vi "CRYResult save as text.vi"(4 "File exists & overwrite (F)":bool, 5 "Excel path":path, 6 "Comment":string, 7 "New/Append":string, 8 "File format":u32, 9 "Format info":T1, 10 "Path":path, 11 "Results stack, flat":string[](array[string])) -> ()   [LabVIEW 2013]
uses:
  Data/CRYData & result stacks global.vi
panel:
  out "error out":errorcluster
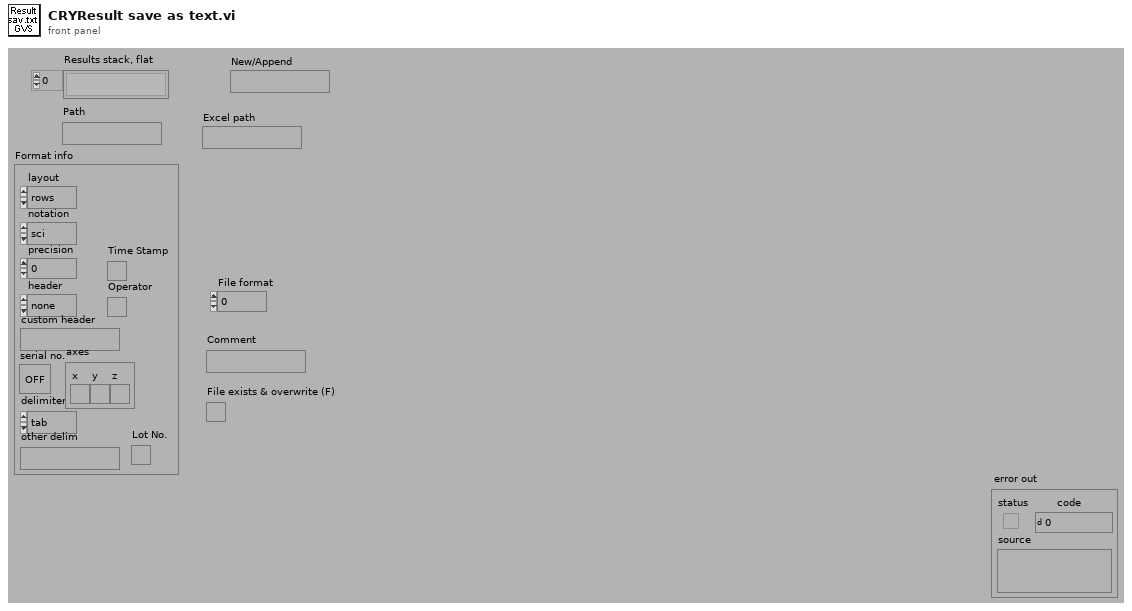
[diagram p1: front panel]
types:
  T1 = cluster{"layout":enum16{"rows", "columns"}, "notation":enum16{"sci", "float"}, "precision":i32, "header":enum16{"none", "standard", "custom"}, "custom header":string, "serial no.":bool, "delimiter":enum16{"tab", "comma", "space", "other"}, "other delim":string, "axes":cluster{"x":bool, "y":bool, "z":bool}, "Lot No.":bool, "Operator":bool, "Time Stamp":bool}
  T2 = typedef "CRYResult Cluster.ctl" = cluster{"Name":string, "Margin":dbl, "unit":string, "Verdict":bool, "Limit":string, "Max/Min":string, "protected":bool, "Step No.":i32, "Test Info":string, "AutoProtect":bool}
  T3 = enum16{"open", "open or create", "create or replace", "create"}
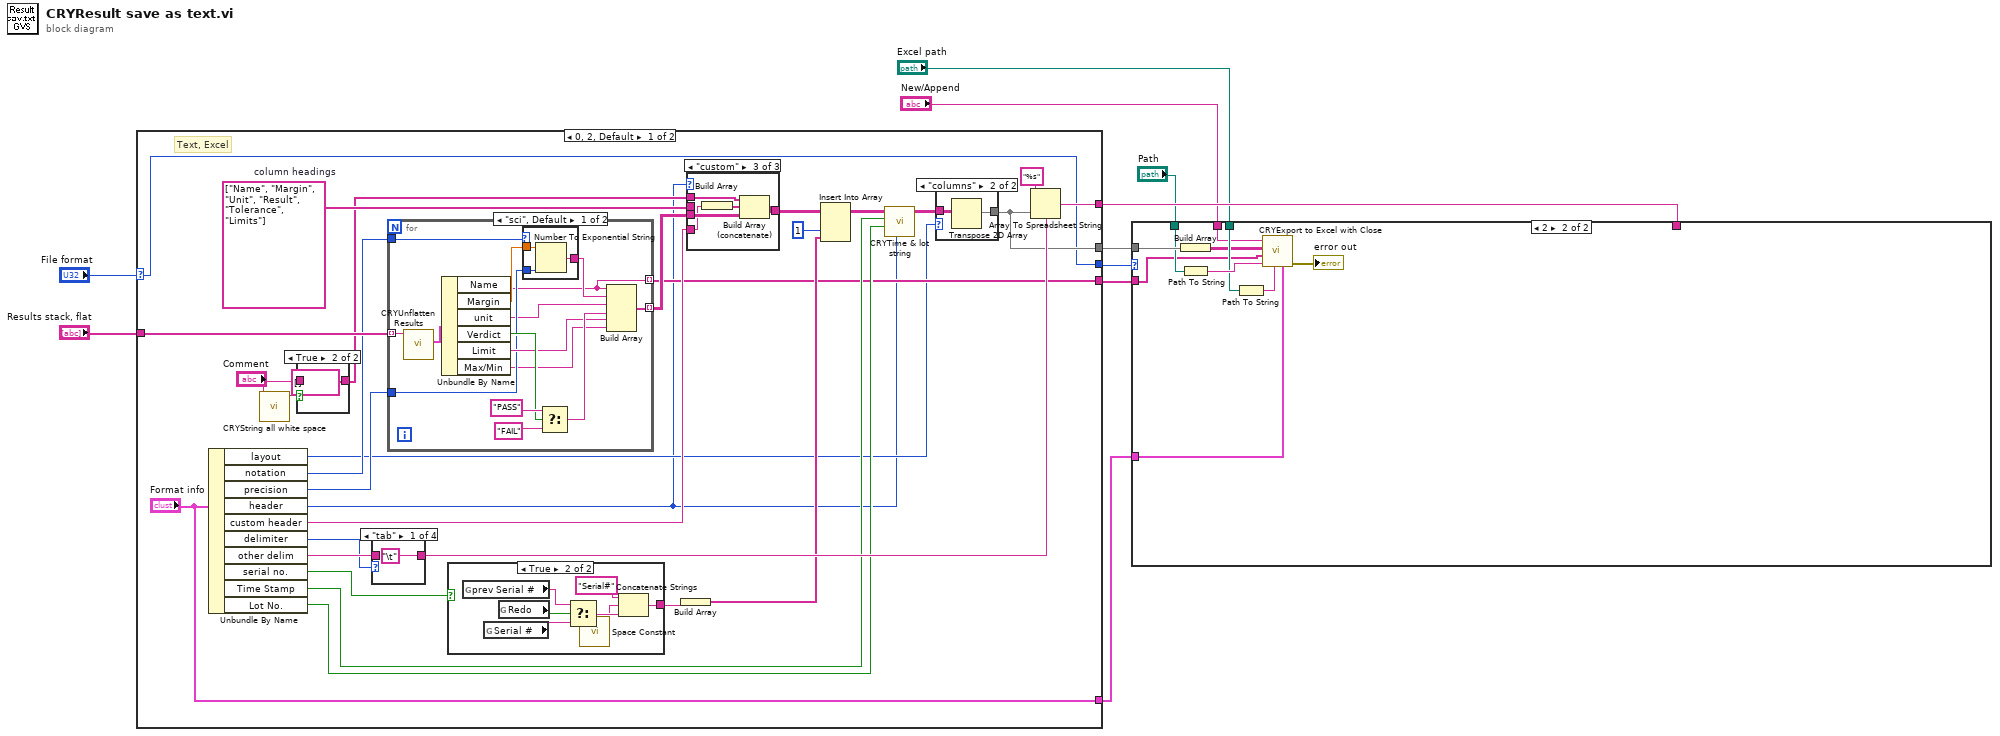
[diagram p0: block diagram]
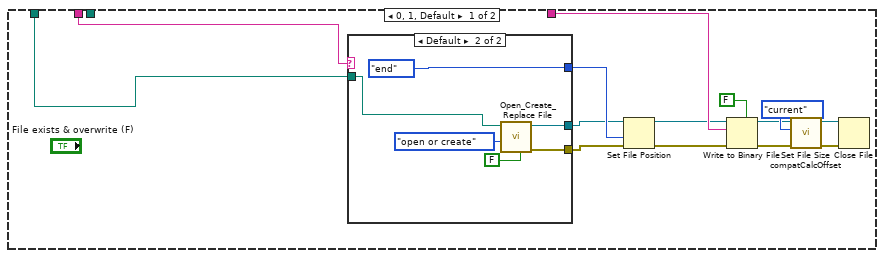
[diagram p2: hidden frame]
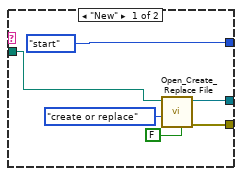
[diagram p3: hidden frame]
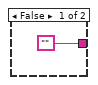
[diagram p4: hidden frame]
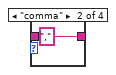
[diagram p5: hidden frame]
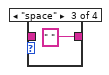
[diagram p6: hidden frame]
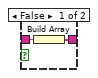
[diagram p8: hidden frame]
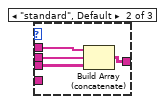
[diagram p10: hidden frame]
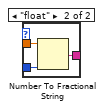
[diagram p12: hidden frame]
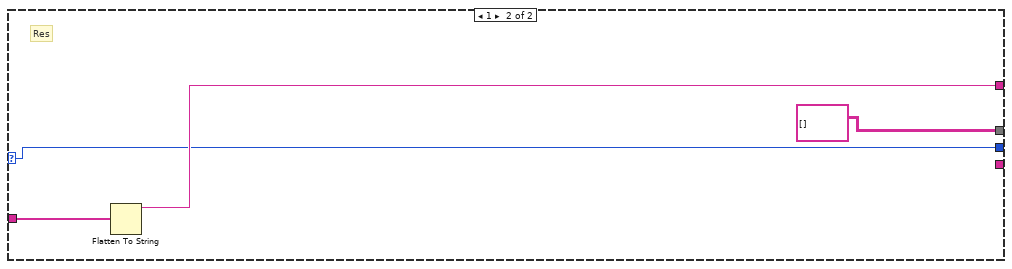
[diagram p13: hidden frame]
diagram:
  n1 = case shown="0, 2, Default" "File format" {
    selector: "File format" -> [w15 w89]
    tunnel: "Results stack, flat" -> [w39 w92]
    tunnel: [w36 w91] -> w9
    tunnel: [w15 w89] -> w4
    tunnel: [w16 string[][] [] ("Table out")] -> w7
    tunnel: [w14 _] -> w3
    tunnel: ["Format info" _] -> w1
    frame 0, 2, Default {
      w38 = string[] ["Name", "Margin", "Unit", "Result", "Tolerance", "Limits"]  # column headings
      # "Text, Excel"
      n2 = Unbundle By Name("Format info") -> ("layout"=w13:enum16{"rows", "columns"}, "notation"=w35:enum16{"sci", "float"}, "precision"=w34:i32, "header"=w11:enum16{"none", "standard", "custom"}, "custom header"=w33:string, "delimiter"=w30:enum16{"tab", "comma", "space", "other"}, "other delim"=w31:string, "serial no."=w26:bool, "Time Stamp"=w25:bool, "Lot No."=w24:bool)
      n3 = call "CRYString all white space.vi"("String"="Comment") -> ("Nothing but white space?"=w27:bool)  [unwired: 10 in]
      n4 = case shown="True" w27 {
        tunnel: "Comment" -> [w53 _]
        tunnel: [w52 string[] []] -> w32
        frame False {
          n5 = Build Array(w53) -> (w52:string[])
        }
        frame True {
        }
      }
      n6 = case shown="\"tab\"" w30 {
        tunnel: w31 -> [_ _ _ w51]
        tunnel: ["\t" "," " " w51] -> w29
        frame "tab" {
        }
        frame "comma" {
        }
        frame "space" {
        }
        frame Default {
        }
      }
      n7 = for {
        tunnel: w39 -> [w69] mode=indexing
        tunnel: w34 -> [w75]
        tunnel: [w77] -> w37 mode=indexing
        tunnel: w35 -> [w74]
        tunnel: [w70] -> w14 mode=indexing
        n8 = call "CRYUnflatten Results.vi"("Unflatten Result"=w69) -> ("Result"=w68:T2)  [unwired: 8 in, 2 out]
        n9 = Unbundle By Name(w68) -> ("Name"=w70:string, "Margin"=w76:dbl, "unit"=w71:string, "Verdict"=w80:bool, "Limit"=w78:string, "Max/Min"=w72:string)
        n10 = case shown="\"sci\", Default" w74 {
          tunnel: w76 -> [w85 w88]
          tunnel: w75 -> [w84 w87]
          tunnel: [w83 w86] -> w73
          frame "sci", Default {
            n11 = Number To Exponential String(number=w85, precision (6)=w84) -> (E-format string=w83:string)  [unwired: 2 out]
          }
          frame "float" {
            n12 = Number To Fractional String(number=w88, precision (6)=w87) -> (F-format string=w86:string)  [unwired: 2 out]
          }
        }
        n13 = Select(t="PASS", s=w80, f="FAIL") -> (s? t:f=w79:string)
        n14 = Build Array(w70, w73, w71, w79, w78, w72) -> (w77:string[])
      }
      n15 = case shown="True" w26 {
        tunnel: ["" w41] -> w21
        frame False {
        }
        frame True {
          n16 = global read "CRYData & result stacks global.vi" "prev Serial #"() -> (w46:string)
          n17 = global read "CRYData & result stacks global.vi" "Serial #"() -> (w47:string)
          n18 = global read "CRYData & result stacks global.vi" "Redo"() -> (w45:bool)
          n19 = Select(t=w46, s=w45, f=w47) -> (s? t:f=w44:string)
          n20 = call <vilib>:"Space Constant.vi"() -> ("String"=w42:string)
          n21 = Concatenate Strings("Serial#" ("string"), w42, w44) -> (w41:string)
        }
      }
      n22 = Build Array(w21) -> (w20:string[])
      n23 = case shown="\"custom\"" w11 {
        tunnel: w38 -> [_ w59 _]
        tunnel: w37 -> [w55 w58 w64]
        tunnel: [w55 w57 w63] -> w23
        tunnel: w33 -> [_ _ w62]
        tunnel: w32 -> [_ w56 w60]
        frame "none" {
        }
        frame "standard", Default {
          n24 = Build Array (concatenate)(w56, w59, w58) -> (w57:string[][])
        }
        frame "custom" {
          n25 = Build Array(w62) -> (w61:string[])
          n26 = Build Array (concatenate)(w60, w61, w64) -> (w63:string[][])
        }
      }
      n27 = Insert Into Array(array=w23, index (col)=1 ("disabled index (col)"), new element=w20) -> (w19:string[][])  [unwired: 1 in]
      n28 = call "CRYTime & lot string.vi"("header"=w11, "Lot No."=w24, "Time Stamp"=w25, "Table in"=w19) -> ("Table out"=w18:string[][])  [unwired: 4 in, 3 out]
      n29 = case shown="\"columns\"" w13 {
        tunnel: w18 -> [w65 w67]
        tunnel: [w65 w66] -> w16
        frame "rows", Default {
        }
        frame "columns" {
          n30 = Transpose 2D Array(2D array=w67) -> (transposed array=w66:string[][])
        }
      }
      n31 = Array To Spreadsheet String(delimiter (Tab)=w29, array=w16, 3:"%s") -> (spreadsheet string=w36:string)
    }
    frame 1 {
      # "Res"
      n32 = Flatten To String(anything=w92) -> (data string=w91:string)  [unwired: 1 in, 4 out]
    }
  }
  n33 = case shown="2" w4 {
    tunnel: w9 -> [w104 _]
    tunnel: w7 -> [_ w131]
    tunnel: "New/Append" -> [w97 w125]
    tunnel: "Path" -> [w95 w130]
    tunnel: w3 -> [_ w123]
    tunnel: "Excel path" -> [_ w128]
    tunnel: w1 -> [_ w122]
    frame 0, 1, Default {
      n34 = case shown="Default" w97 {
        tunnel: [enum16{"start", "end", "current"}."start" ("from (0:start)") enum16{"start", "end", "current"}."end" ("from (0:start)")] -> w96
        tunnel: w95 -> [w112 w118]
        tunnel: [w111 w117] -> w94
        tunnel: [w110 w116] -> w93
        frame "New" {
          n35 = call <vilib>:"Open_Create_Replace File.vi"("advisory dialog? (display:T)"=FALSE, "function (open:0)"=T3."create or replace", "file path"=w112) -> ("error out"=w110:errorcluster, "refnum"=w111:refnum<file>)  [unwired: 4 in, 3 out]
        }
        frame Default {
          n36 = call <vilib>:"Open_Create_Replace File.vi"("advisory dialog? (display:T)"=FALSE, "function (open:0)"=T3."open or create", "file path"=w118) -> ("error out"=w116:errorcluster, "refnum"=w117:refnum<file>)  [unwired: 4 in, 3 out]
        }
      }
      n37 = Set File Position(refnum=w94, from (0:start)=w96, error in=w93) -> (refnum out=w99:refnum<file>, error out=w98:errorcluster)  [unwired: 1 in]
      n38 = Write to Binary File(file (use dialog)=w99, data=w104, error in=w98, 5:FALSE ("预置数组或字符串大小？(T)")) -> (refnum out=w107:refnum<file>, error out=w108:errorcluster)  [unwired: 3 out]
      n39 = call <vilib>:"compatCalcOffset.vi"("error in"=w108, "pos mode (0:1)"=enum16{"start", "end", "current"}."current", "refnum"=w107) -> ("error out"=w102:errorcluster, "offset"=w101:i32, "dup refnum"=w100:refnum<file>)  [unwired: 1 in, 5 out]
      n40 = Set File Size(4:w102, 6:w101, 7:w100) -> (0:w105:errorcluster, 3:w106:refnum<file>)
      n41 = Close File(refnum=w106, error in=w105) -> ()  [unwired: 2 out]
    }
    frame 2 {
      n42 = Build Array(w131) -> (w124:string[][][])
      n43 = Path To String(path=w130) -> (string=w129:string)
      n44 = Path To String(path=w128) -> (string=w126:string)
      n45 = call "CRYExport to Excel with Close.vi"("Format info"=w122, "ExcelPath"=w126, "FilePath"=w129, "Sheet Names"=w123, "Data"=w124, "New/Append"=w125) -> ("error out"=→"error out":errorcluster)  [unwired: 5 in]
    }
  }
